vi "Open ITC.vi"(8 "error in (no error)":errorcluster, 11 "Instrument.Oxford1820 in":refnum<class "Instrument.Oxford1820.lvclass">) -> (0 "error out":errorcluster, 3 "Instrument.Oxford1820 out":refnum<class "Instrument.Oxford1820.lvclass">)   [LabVIEW 2019, in "Instrument.Oxford1820.lvclass"]
uses:
  Instrument.Oxford1820.lvclass
  <instrlib>/Mercury iXX/Public/Controls/Comms Transport Layer.ctl
  Instrument.Oxford1820.lvclass/Instrument.Oxford1820.ctl
  <instrlib>/Mercury iXX/Public/Libraries/System/Open/Open System.vi
  <instrlib>/Mercury iXX/Public/Libraries/System/Read/Catalogue (Read).vi
  <instrlib>/Mercury iXX/Mercury iXX.lvlib
  <instrlib>/Mercury iXX/Public/Libraries/System.lvlib
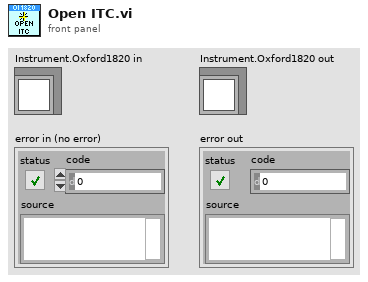
[diagram p1: front panel]
types:
  T1 = typedef "Mercury iXX.lvlib/Comms Transport Layer.ctl" = enum16{"Ethernet TCP/IP", "USB", "ISOBus - RS-232", "GPIB"}
  T2 = typedef "Mercury iXX.lvlib/Mercury Reference.ctl" = cluster{"Comms":refnum<visa-resource-name>, "Device ID":string[], "Comms Layer":T1, "Command":string, "Query reference":T3}
  T3 = typedef "Mercury iXX.lvlib/Query Dynamic Reference.ctl" = refnum<vi>
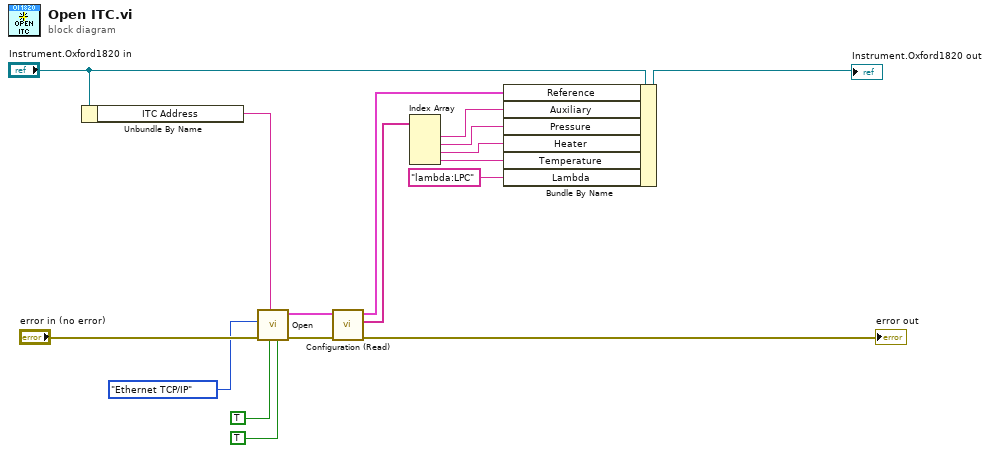
[diagram p0: block diagram]
diagram:
  n1 = Unbundle By Name("Instrument.Oxford1820 in") -> ("ITC Address"=w3:string)
  n2 = call-poly <instrlib>:"Open.vi"("Clear Previous Connections (False)"=TRUE, "ID Query (True)"=TRUE, "IP Address"=w3, "error in (no error)"="error in (no error)", "Comms Layer"=Comms_Transport_Layer."Ethernet TCP/IP") -> ("error out"=w15:errorcluster, "Mercury Reference Out"=w14:T2)  [unwired: 2 in, 3 out]
  n3 = call-poly <instrlib>:"Configuration (Read).vi"("error in"=w15, "Mercury Reference In"=w14) -> ("error out"=→"error out":errorcluster, "Devices"=w9:string[], "Mercury Reference Out"=w1:T2)  [unwired: 1 in, 6 out]
  n4 = Index Array(array=w9) -> (element #1=w10:string, element #2=w11:string, element #3=w12:string, element #4=w13:string)  [unwired: 4 in]
  n5 = Bundle By Name(cluster="Instrument.Oxford1820 in", "Reference"=w1, "Auxiliary"=w10, "Pressure"=w11, "Heater"=w12, "Temperature"=w13, "Lambda"="lambda:LPC" ("Device Identifier")) -> (→"Instrument.Oxford1820 out":refnum<class "Instrument.Oxford1820.lvclass">)
